vi "Shift_Register.vi"() -> ()   [LabVIEW 2015]
panel:
  out "Shift Value":dbl
  out "Sum":dbl
  in  "?":dbl
  in  "milliseconds to wait":u32=100
  out "Waveform Graph":i32[](graph)=[0, 1, 2, 3, 4, 5, 6, 7, 8, 9]
  out "Final Value":dbl=9.0
  out "iteration":dbl=9.0
  in  "Number of\nIterations":i32=10
  # "External Input"
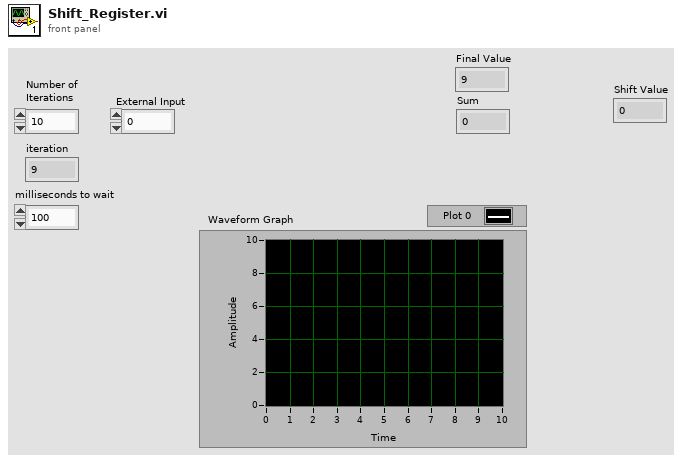
[diagram p1: front panel]
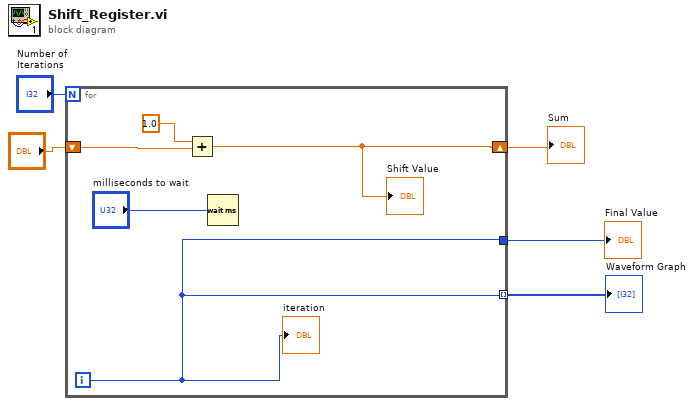
[diagram p0: block diagram]
diagram:
  n1 = for {
    N: "Number of\nIterations" -> [_]
    tunnel: [w10] -> w3 mode=indexing
    tunnel: [w10] -> w4
    shift-right: [w6] -> w1
    shift-left: "?" -> [w7]
    i -> [w10]
    n2 = Add(x=1.0, y=w7) -> (x+y=w6:dbl)
    "Shift Value" <- w6
    n3 = Wait (ms)(milliseconds to wait="milliseconds to wait") -> ()  [unwired: 1 out]
    "iteration" <- w10
  }
  "Final Value" <- w4
  "Waveform Graph" <- w3
  "Sum" <- w1
